vi "sub_DTMF_Quantize_BitEncoding.vi"(0 "signal":dbl[](array[numeric]), 5 "L":u16=16 min=2, 9 "xmin":dbl=-1.0, 11 "xmax":dbl=1.0, 12 "GrayCode":bool) -> (4 "TXbitStream":i32[](array[numeric]), 6 "quants":dbl[](array[numeric]), 8 "qmin":dbl, 10 "qmax":dbl, 15 "bitLength":i32)   [LabVIEW 2011]
uses:
  <vilib>/imath/engines/lvmath2/RunTimeEngine/ErrorHandling/NIMS_Finalize Error.vi
  <vilib>/imath/engines/lvmath2/RunTimeEngine/VariableToken/NIMS_VariableToken_CondDefined.vi
  <instcachedir>/0/NIMS_VariableToken_CondDefined_D30D2F4D3CE04567BC79CC35D27951F7.lvgen/NIMS_VariableToken_CondDefined_D30D2F4D3CE04567BC79CC35D27951F7_005.vi
  <vilib>/imathl/engines/lvmath/Functions/Error Handling/Create Error.vi
  <vilib>/imath/engines/lvmath2/RunTimeEngine/NodeEndStatement/NIMS_NodeEndStatement_Output.vi
  <instcachedir>/0/NIMS_NodeEndStatement_Output_53EC0D466D134D7ABD903AC30B43404B.lvgen/NIMS_NodeEndStatement_Output_53EC0D466D134D7ABD903AC30B43404B_012.vi
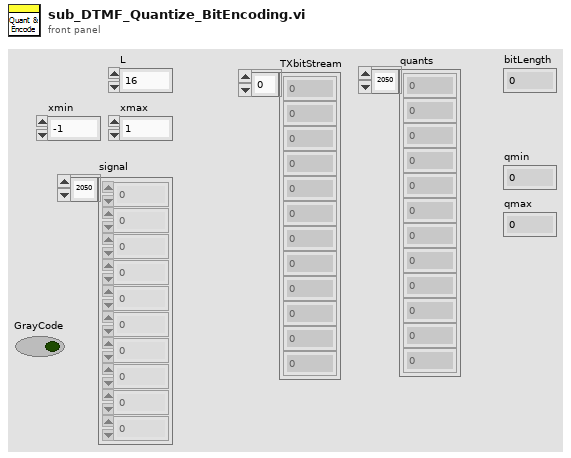
[diagram p1: front panel]
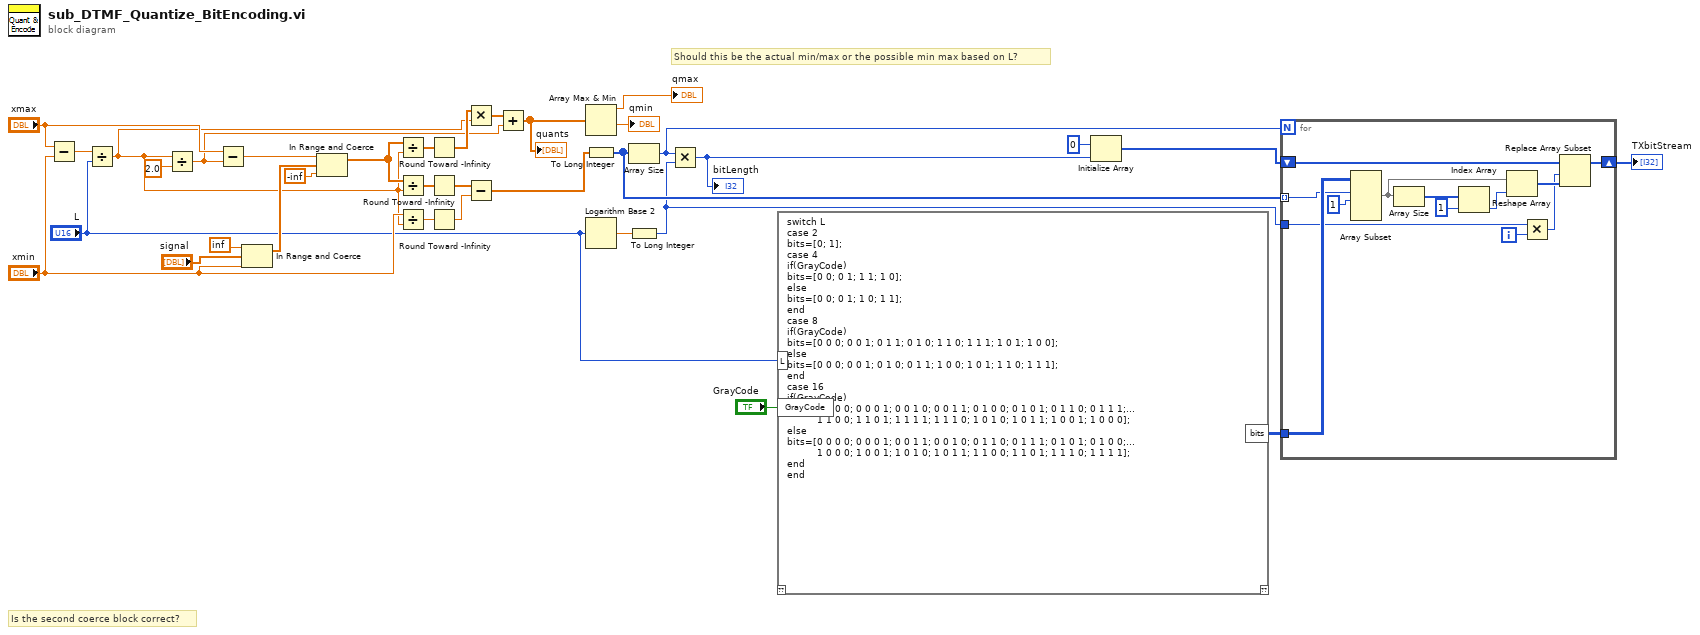
[diagram p0: block diagram]
diagram:
  # "Should this be the actual min/max or the possible min max based on L?"
  # "Is the second coerce block correct?"
  n1 = Subtract(x="xmax", y="xmin") -> (x-y=w34:dbl)
  n2 = Divide(x=w34, y="L") -> (x/y=w18:dbl)
  n3 = Divide(x=w18, y=2.0) -> (x/y=w16:dbl)
  n4 = Subtract(x="xmax", y=w16) -> (x-y=w24:dbl)
  n5 = In Range and Coerce(upper limit=inf, x="signal", lower limit="xmin") -> (coerced(x)=w27:dbl[])  [unwired: 1 out]
  n6 = In Range and Coerce(upper limit=w24, x=w27, lower limit=-inf) -> (coerced(x)=w21:dbl[])  [unwired: 1 out]
  n7 = Divide(x=w21, y=w18) -> (x/y=w20:dbl[])
  n8 = Divide(x=w21, y=w18) -> (x/y=w33:dbl[])
  n9 = Divide(x="xmin", y=w18) -> (x/y=w31:dbl)
  n10 = Round Toward -Infinity(1:w20) -> (0:w19:dbl[])
  n11 = Round Toward -Infinity(1:w33) -> (0:w32:dbl[])
  n12 = Round Toward -Infinity(1:w31) -> (0:w30:dbl)
  n13 = Multiply(x=w19, y=w18) -> (x*y=w17:dbl[])
  n14 = Subtract(x=w32, y=w30) -> (x-y=w1:dbl[])
  n15 = Add(x=w17, y=w16) -> (x+y=w15:dbl[])
  "quants" <- w15
  n16 = Array Max & Min(array=w15) -> (max value=→"qmax":dbl, min value=→"qmin":dbl)  [unwired: 2 out]
  n17 = To Long Integer(number=w1) -> (32bit integer=w6:i32[])
  n18 = Logarithm Base 2(1:"L") -> (0:w7:dbl)
  n19 = Array Size(array=w6) -> (size(s)=w4:i32)
  n20 = To Long Integer(number=w7) -> (32bit integer=w3:i32)
  n21 = Multiply(x=w4, y=w3) -> (x*y=w2:i32)
  "bitLength" <- w2
  n22 = mathscript code="switch L\ncase 2\nbits=[0; 1];\ncase 4\nif(GrayCode)\nbits=[0 0; 0 1; 1 1; 1 0];\nelse\nbits=[0 0; 0 1; 1 0; 1 1];\nend\ncase 8\nif(GrayCode)\nbits=[0 0 0; 0 0 1; 0 1 1; 0 1 0; 1 1 0; 1 1 1; 1 0 1; 1 0 0];\nelse\nbits=[0 0 0; 0 0 1; 0 1 0; 0 1 1; 1 0 0; 1 0 1; 1 1 0; 1 1 1];\nend\ncase 16\nif(GrayCode)\nbits=[0 0 0 0; 0 0 0 1; 0 0 1 0; 0 0 1 1; 0 1 0 0; 0 1 0 1; 0 1 1 0; 0 1 1 1;...\n          1 1 0 0; 1 1 0 1; 1 1 1 1; 1 1 1 0; 1 0 1 0; 1 0 1 1; 1 0 0 1; 1 0 0 0];\nelse\nbits=[0 0 0 0; 0 0 0 1; 0 0 1 1; 0 0 1 0; 0 1 1 0; 0 1 1 1; 0 1 0 1; 0 1 0 0;...\n          1 0 0 0; 1 0 0 1; 1 0 1 0; 1 0 1 1; 1 1 0 0; 1 1 0 1; 1 1 1 0; 1 1 1 1];\nend\nend"("L"="L", "GrayCode"="GrayCode") -> ("bits"=w9:i32[][])  [unwired: 1 in, 1 out]
  n23 = Initialize Array(0 ("element"), w2) -> (w10:i32[])
  n24 = for {
    N: w4 -> [_]
    tunnel: w6 -> [w35] mode=indexing
    shift-right: [w40] -> w5
    shift-left: w10 -> [w44]
    tunnel: w9 -> [w46]
    tunnel: w3 -> [w42]
    i -> [w43]
    n25 = Array Subset(array=w46, index (row)=w35, length (row)=1 ("length")) -> (w39:i32[][])  [unwired: 2 in]
    n26 = Array Size(array=w39) -> (size(s)=w38:i32[])
    n27 = Index Array(array=w38, index=1) -> (element=w37:i32)
    n28 = Reshape Array(w39, w37) -> (w45:i32[])
    n29 = Multiply(x=w42, y=w43) -> (x*y=w41:i32)
    n30 = Replace Array Subset(array=w44, new element=w45, index=w41) -> (w40:i32[])
  }
  "TXbitStream" <- w5
